vi "Integration Simpsons Rule (1 Ch).vi"(8 "error in (no error)":errorcluster, 10 "Integration Type":T1(ring), 11 "Waveform":waveform(sgl)) -> (0 "error out":errorcluster, 2 "Integrated Waveform":waveform(sgl))   [LabVIEW 2017, in "VibrationAnalysisFunctions.lvlib"]
uses:
  <vilib>/addons/InsightCM/Utilities/Analysis/Vibration/VibrationAnalysisFunctions.lvlib
  <vilib>/Analysis/2dsp.llb/Integral Method.ctl
  <vilib>/Analysis/NI_AALPro.lvlib
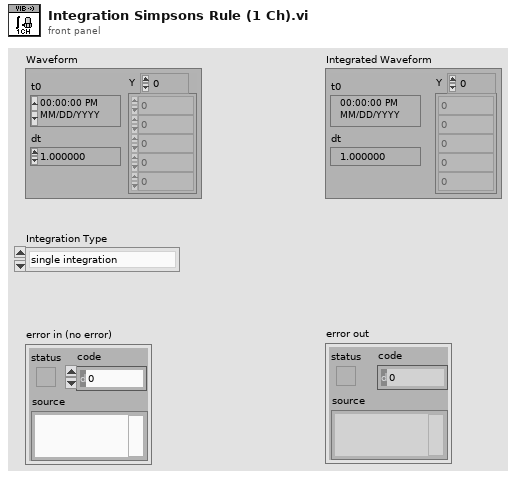
[diagram p1: front panel]
types:
  T1 = enum16{"single integration", "double integration", "single differentiation", "double differentiation", "none"}
  T2 = typedef "NI_AALPro.lvlib/Integral Method.ctl" = i32
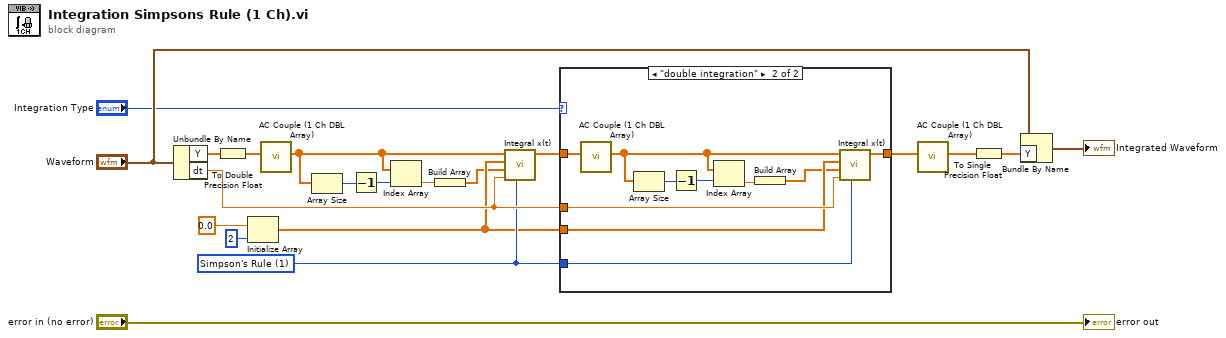
[diagram p0: block diagram]
diagram:
  w12 = T2 1 items=["Trapezoidal Rule", "Simpson's Rule", "Simpson's 3/8 Rule", "Bode Rule"] ("integration method")
  n1 = Unbundle By Name("Waveform") -> ("Y"=w16:sgl[], "dt"=w13:dbl)
  n2 = To Double Precision Float(number=w16) -> (double precision float=w15:dbl[])
  n3 = Initialize Array(0.0 ("dt"), 2 ("dimension size")) -> (w6:dbl[])
  n4 = call <vilib>:"AC Couple (1 Ch DBL Array).vi"("Signal"=w15) -> ("AC Coupled"=w5:dbl[])  [unwired: 8 in, 2 out]
  n5 = Array Size(array=w5) -> (size(s)=w4:i32)
  n6 = Decrement(x=w4) -> (x-1=w3:i32)
  n7 = Index Array(array=w5, index=w3) -> (element=w2:dbl)
  n8 = Build Array(w2) -> (w1:dbl[])
  n9 = call <vilib>:"Integral x(t).vi"("integration method"=w12, "dt"=w13, "Final Condition"=w1, "Initial Condition"=w6, "X"=w5) -> ("Integral X"=w17:dbl[])  [unwired: 5 in, 1 out]
  n10 = case shown="\"double integration\"" "Integration Type" {
    tunnel: [w21 w28] -> w10
    tunnel: w17 -> [w21 w31]
    tunnel: w6 -> [_ w27]
    tunnel: w13 -> [_ w30]
    tunnel: w12 -> [_ w29]
    frame "single integration", Default {
    }
    frame "double integration" {
      n11 = call <vilib>:"AC Couple (1 Ch DBL Array).vi"("Signal"=w31) -> ("AC Coupled"=w23:dbl[])  [unwired: 8 in, 2 out]
      n12 = Array Size(array=w23) -> (size(s)=w26:i32)
      n13 = Decrement(x=w26) -> (x-1=w25:i32)
      n14 = Index Array(array=w23, index=w25) -> (element=w24:dbl)
      n15 = Build Array(w24) -> (w22:dbl[])
      n16 = call <vilib>:"Integral x(t).vi"("integration method"=w29, "dt"=w30, "Final Condition"=w22, "Initial Condition"=w27, "X"=w23) -> ("Integral X"=w28:dbl[])  [unwired: 5 in, 1 out]
    }
  }
  n17 = call <vilib>:"AC Couple (1 Ch DBL Array).vi"("Signal"=w10) -> ("AC Coupled"=w9:dbl[])  [unwired: 8 in, 2 out]
  n18 = To Single Precision Float(number=w9) -> (single precision float=w8:sgl[])
  n19 = Bundle By Name(cluster="Waveform", "Y"=w8) -> (→"Integrated Waveform":waveform(sgl))
  "error out" <- "error in (no error)"
